vi "Teleop.vi"(10 "Match Info":T1={"Autonomous Elapsed Seconds"=0.0, "TeleOp Elapsed Seconds"=0.0, "Disabled Elapsed Seconds"=0.0, "Visited Autonomous"=FALSE, "Visited TeleOp"=FALSE, "Visited Disabled"=FALSE, "Autonomous Settings"={"Autonomous Style"=enum."Independent", "VI Refnum"=refnum}}, 11 "Call Context":T2) -> ()   [LabVIEW 2018]
doc: "This VI is called for each enabled TeleOp packet received from the DS. It is typically used to read from joysticks and other inputs and update I/O or setpoints for timed control loops. It should complete and return within 20 milliseconds or risk missing DS packets."
uses:
  <vilib>/Rock Robotics/WPI/DriverStation/WPI_DriverStationDerivedRobotMode.ctl
  <vilib>/Rock Robotics/WPI/DriverStation/WPI_DriverStationMatch Info.ctl
  Framework/Robot Global Data.vi
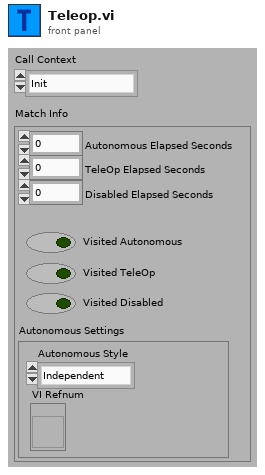
[diagram p1: front panel]
types:
  T1 = typedef "WPI_DriverStationMatch Info.ctl" = cluster{"Autonomous Elapsed Seconds":dbl, "TeleOp Elapsed Seconds":dbl, "Disabled Elapsed Seconds":dbl, "Visited Autonomous":bool, "Visited TeleOp":bool, "Visited Disabled":bool, "Autonomous Settings":cluster{"Autonomous Style":enum16{"Iterative", "Independent"}, "VI Refnum":refnum<vi>}}
  T2 = typedef "WPI_DriverStationDerivedRobotMode.ctl" = enum16{"Init", "Execute", "Stop"}
  T3 = typedef "Command Status Info.ctl" = cluster{"Name":string, "Status":T4, "notifier out":T5}
  T4 = typedef "Completion Status.ctl" = enum16{"Successful", "Aborted", "Incomplete"}
  T5 = typedef "Completion Notifier.ctl" = refnum<notifier>
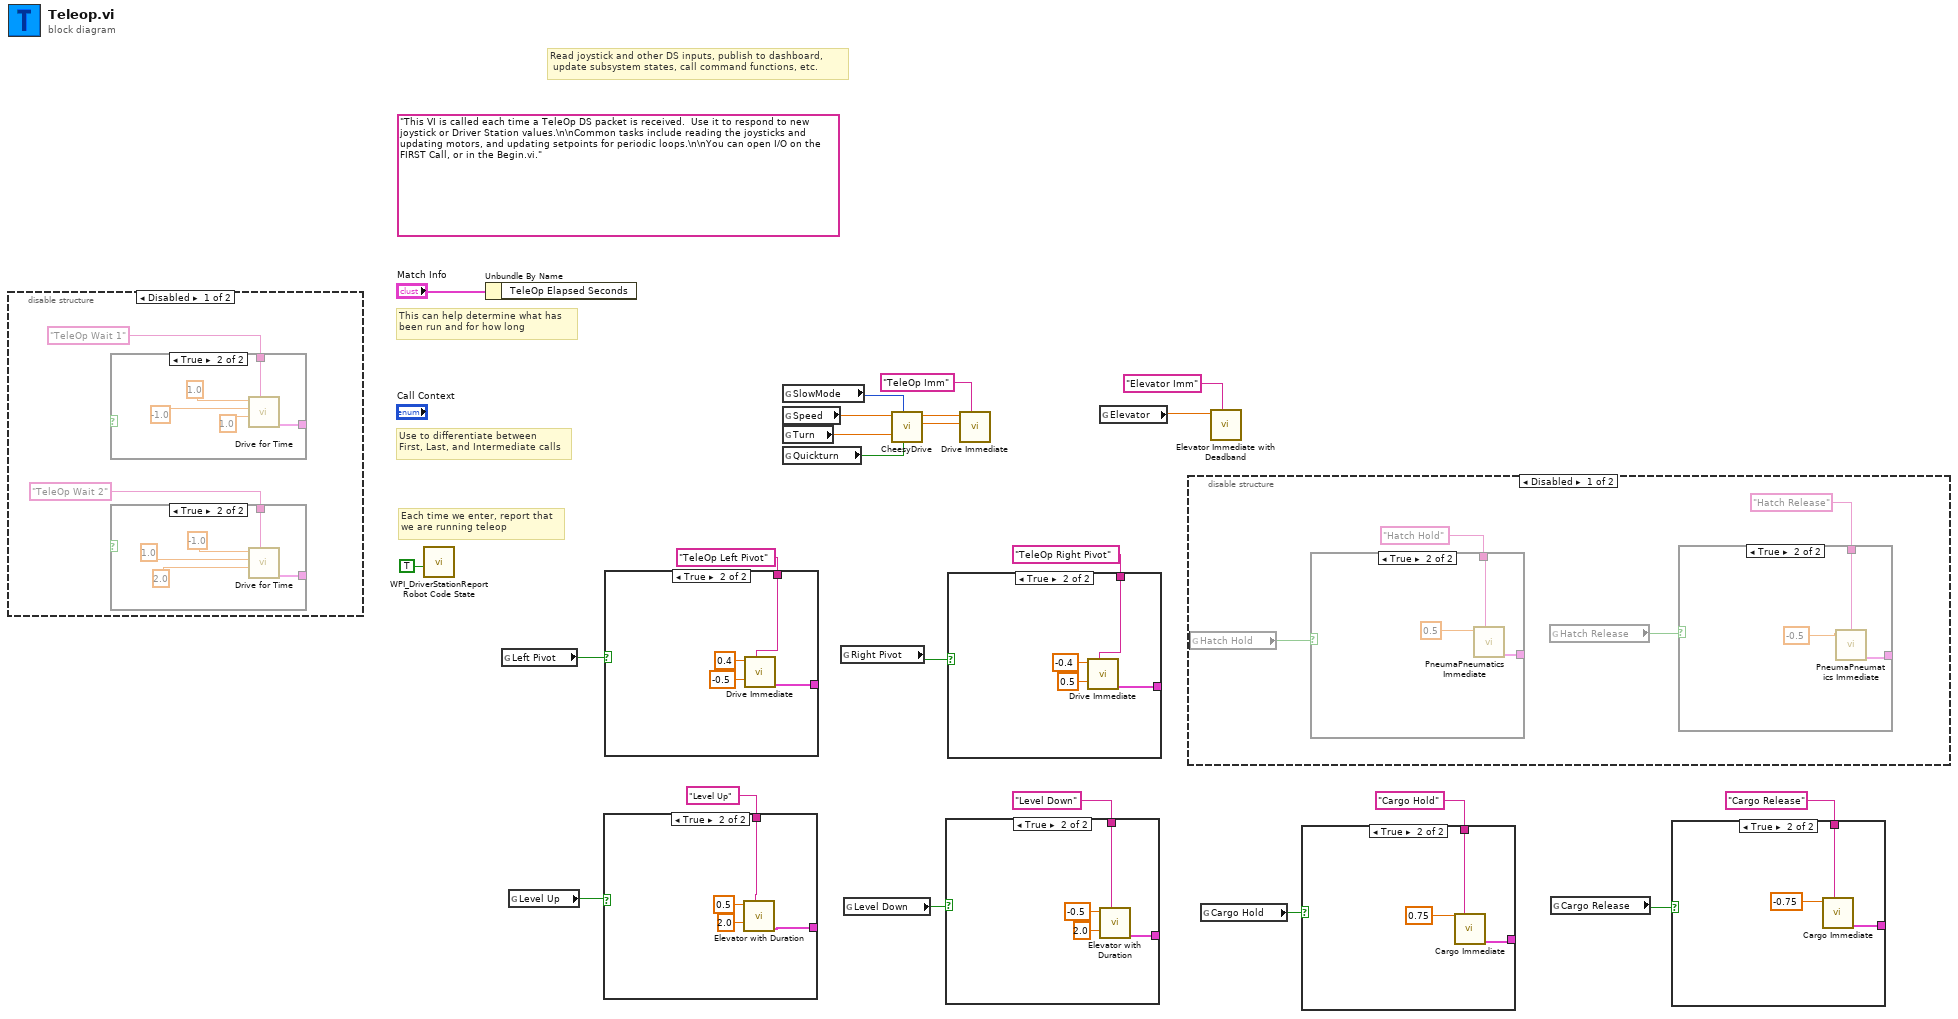
[diagram p0: block diagram]
diagram:
  (unwired) "This VI is called each time a TeleOp DS packet is received.  Use it to respond to new joystick or Driver Station values.\n\nCommon tasks include reading the joysticks and updating motors, and updating setpoints for periodic loops.\n\nYou can open I/O on the FIRST Call, or in the Begin.vi."
  # "Read joystick and other DS inputs, publish to dashboard,\n update subsystem states, call command functions, etc."
  # "Each time we enter, report that\nwe are running teleop"
  # "Use to differentiate between\nFirst, Last, and Intermediate calls"
  # "This can help determine what has\nbeen run and for how long"
  n1 = disable-structure shown="Disabled" {
    frame Disabled {
      n2 = case shown="True" w25 {
        tunnel: [_ w36] -> _
        tunnel: "TeleOp Wait 1" ("Description") -> [_ w35]
        frame False {
        }
        frame True {
          n3 = call "Drive for Time.vi"("Description"=w35, "Seconds"=1.0, "Right Speed"=-1.0, "Left Speed"=1.0) -> ("Command Info Out"=w36:T3)  [unwired: 7 in]
        }
      }
      n4 = case shown="True" w24 {
        tunnel: [_ w30] -> _
        tunnel: "TeleOp Wait 2" ("Description") -> [_ w29]
        frame False {
        }
        frame True {
          n5 = call "Drive for Time.vi"("Description"=w29, "Seconds"=2.0, "Right Speed"=1.0, "Left Speed"=-1.0) -> ("Command Info Out"=w30:T3)  [unwired: 7 in]
        }
      }
    }
    frame Enabled {
    }
  }
  n6 = call <vilib>:"WPI_DriverStationReport Robot Code State.vi"("TeleOp"=TRUE ("Autonomous")) -> ()  [unwired: 10 in, 1 out]
  n7 = Unbundle By Name("Match Info") -> ()  [unwired: 1 out]
  n8 = global read "Robot Global Data.vi" "Left Pivot"() -> (w12:bool)
  n9 = global read "Robot Global Data.vi" "Level Up"() -> (w8:bool)
  n10 = case shown="True" w8 {
    tunnel: [_ w41] -> _
    tunnel: "Level Up" ("Description") -> [_ w40]
    frame False {
    }
    frame True {
      n11 = call "Elevator with Duration.vi"("Description"=w40, "Duration (s)"=2.0, "Setpoint"=0.5) -> ("Command Info Out"=w41:T3)  [unwired: 8 in]
    }
  }
  n12 = case shown="True" w12 {
    tunnel: [_ w43] -> _
    tunnel: "TeleOp Left Pivot" ("Description") -> [_ w42]
    frame False {
    }
    frame True {
      n13 = call "Drive Immediate.vi"("Description"=w42, "Right Setpoint"=-0.5, "Left Setpoint"=0.4) -> ("Command Info Out"=w43:T3)  [unwired: 8 in]
    }
  }
  n14 = global read "Robot Global Data.vi" "SlowMode"() -> (w11:u32)
  n15 = global read "Robot Global Data.vi" "Speed"() -> (w18:dbl)
  n16 = global read "Robot Global Data.vi" "Turn"() -> (w17:dbl)
  n17 = global read "Robot Global Data.vi" "Quickturn"() -> (w16:bool)
  n18 = global read "Robot Global Data.vi" "Right Pivot"() -> (w13:bool)
  n19 = global read "Robot Global Data.vi" "Level Down"() -> (w7:bool)
  n20 = call "CheesyDrive.vi"("Quickturn"=w16, "SlowMode"=w11, "Wheel"=w17, "Throttle"=w18) -> ("Right PWM"=w19:dbl, "Left PWM"=w20:dbl)  [unwired: 6 in]
  n21 = case shown="True" w7 {
    tunnel: "Level Down" ("Description") -> [_ w49]
    tunnel: [_ w48] -> _
    frame False {
    }
    frame True {
      n22 = call "Elevator with Duration.vi"("Description"=w49, "Duration (s)"=2.0, "Setpoint"=-0.5) -> ("Command Info Out"=w48:T3)  [unwired: 8 in]
    }
  }
  n23 = case shown="True" w13 {
    tunnel: [_ w51] -> _
    tunnel: "TeleOp Right Pivot" ("Description") -> [_ w50]
    frame False {
    }
    frame True {
      n24 = call "Drive Immediate.vi"("Description"=w50, "Right Setpoint"=0.5, "Left Setpoint"=-0.4) -> ("Command Info Out"=w51:T3)  [unwired: 8 in]
    }
  }
  n25 = call "Drive Immediate.vi"("Description"="TeleOp Imm", "Right Setpoint"=w19, "Left Setpoint"=w20) -> ()  [unwired: 8 in, 1 out]
  n26 = global read "Robot Global Data.vi" "Elevator"() -> (w2:dbl)
  n27 = disable-structure shown="Disabled" {
    frame Disabled {
      n28 = global read "Robot Global Data.vi" "Hatch Hold"() -> (w54:bool)
      n29 = case shown="True" w54 {
        tunnel: "Hatch Hold" ("Description") -> [_ w62]
        tunnel: [_ w61] -> _
        frame False {
        }
        frame True {
          n30 = call "PneumaPneumatics Immediate.vi"("Description"=w62, "Setpoint"=0.5 ("Left Setpoint")) -> ("Command Info Out"=w61:T3)  [unwired: 9 in]
        }
      }
      n31 = global read "Robot Global Data.vi" "Hatch Release"() -> (w55:bool)
      n32 = case shown="True" w55 {
        tunnel: "Hatch Release" ("Description") -> [_ w59]
        tunnel: [_ w58] -> _
        frame False {
        }
        frame True {
          n33 = call "PneumaPneumatics Immediate.vi"("Description"=w59, "Setpoint"=-0.5 ("Left Setpoint")) -> ("Command Info Out"=w58:T3)  [unwired: 9 in]
        }
      }
    }
    frame Enabled {
    }
  }
  n34 = global read "Robot Global Data.vi" "Cargo Hold"() -> (w4:bool)
  n35 = call "Elevator Immediate with Deadband.vi"("Description"="Elevator Imm", "Setpoint"=w2) -> ()  [unwired: 9 in, 1 out]
  n36 = case shown="True" w4 {
    tunnel: [_ w66] -> _
    tunnel: "Cargo Hold" ("Description") -> [_ w65]
    frame False {
    }
    frame True {
      n37 = call "Cargo Immediate.vi"("Description"=w65, "Setpoint"=0.75 ("Left Setpoint")) -> ("Command Info Out"=w66:T3)  [unwired: 9 in]
    }
  }
  n38 = global read "Robot Global Data.vi" "Cargo Release"() -> (w3:bool)
  n39 = case shown="True" w3 {
    tunnel: [_ w69] -> _
    tunnel: "Cargo Release" ("Description") -> [_ w67]
    frame False {
    }
    frame True {
      n40 = call "Cargo Immediate.vi"("Description"=w67, "Setpoint"=-0.75 ("Left Setpoint")) -> ("Command Info Out"=w69:T3)  [unwired: 9 in]
    }
  }
